vi "Geometric_Data.vi"() -> ()   [LabVIEW 2021]
panel:
  in  "cube length":dbl
  out "Volume 3":dbl
  out "L.S.A 2":dbl
  out "T.S.A 3":dbl
  out "On/Off":bool
  in  "stop 3":bool
  in  "circular cone arm length":dbl
  in  "circular cone radius":dbl
  in  "circular cone hieght":dbl
  out "Volume 2":dbl
  out "L.S.A":dbl
  out "T.S.A 2":dbl
  out "On/Off":bool
  in  "stop":bool
  in  "stop":bool
  out "On/Off":bool
  out "T.S.A":dbl
  out "L.S.A":dbl
  out "Volume":dbl
  in  "Cylinder Hieght":dbl
  in  "Cylinder Radius":dbl
  # "Cylinder"
  # "Circular Cone"
  # "Cube"
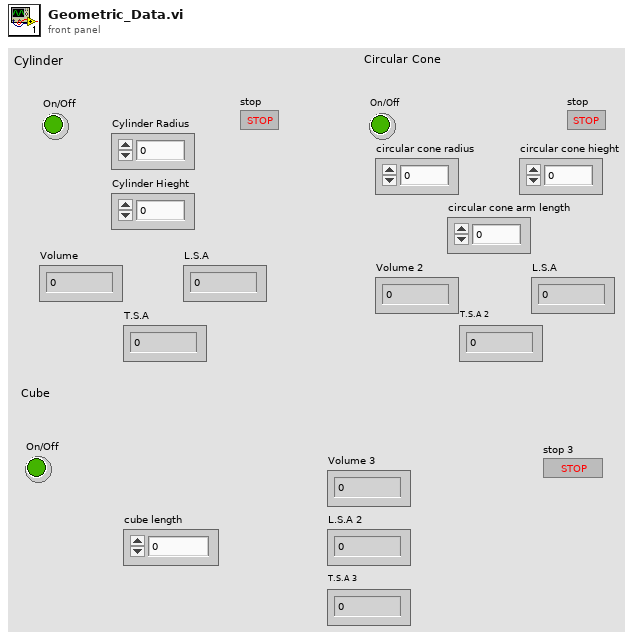
[diagram p1: front panel]
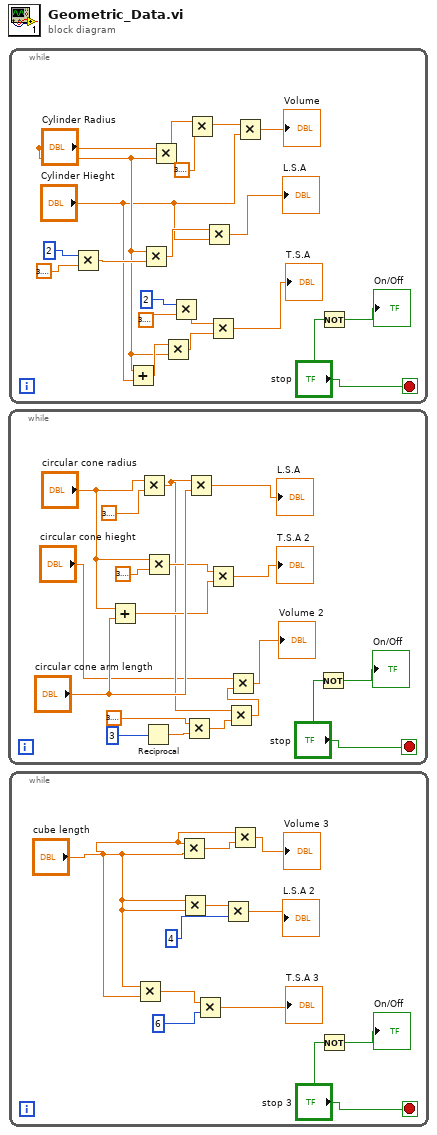
[diagram p0: block diagram]
diagram:
  n1 = while {
    stop <- "stop" stop-if-true
    n2 = Add(x="circular cone radius", y="circular cone arm length") -> (x+y=w10:dbl)
    n3 = Multiply(x="circular cone radius", y=3.141592653589793) -> (x*y=w4:dbl)
    n4 = Reciprocal(x=3) -> (1/x=w6:dbl)
    n5 = Multiply(x="circular cone radius", y=3.141592653589793) -> (x*y=w11:dbl)
    n6 = Multiply(x=3.141592653589793, y=w6) -> (x*y=w5:dbl)
    n7 = Multiply(x=w4, y="circular cone arm length") -> (x*y=→"L.S.A":dbl)
    n8 = Multiply(x=w11, y=w10) -> (x*y=→"T.S.A 2":dbl)
    n9 = Multiply(x=w4, y=w5) -> (x*y=w3:dbl)
    n10 = Multiply(x="circular cone hieght", y=w3) -> (x*y=→"Volume 2":dbl)
    n11 = Not(x="stop") -> (.not. x?=→"On/Off":bool)
  }
  n12 = while {
    stop <- "stop" stop-if-true
    n13 = Multiply(x=2, y=3.141592653589793) -> (x*y=w33:dbl)
    n14 = Add(x="Cylinder Radius", y="Cylinder Hieght") -> (x+y=w30:dbl)
    n15 = Multiply(x="Cylinder Radius", y=w33) -> (x*y=w32:dbl)
    n16 = Multiply(x="Cylinder Radius", y="Cylinder Radius") -> (x*y=w37:dbl)
    n17 = Multiply(x=w30, y="Cylinder Radius") -> (x*y=w25:dbl)
    n18 = Multiply(x=2, y=3.141592653589793) -> (x*y=w26:dbl)
    n19 = Multiply(x=w37, y=3.141592653589793) -> (x*y=w20:dbl)
    n20 = Multiply(x=w32, y="Cylinder Hieght") -> (x*y=→"L.S.A":dbl)
    n21 = Multiply(x=w26, y=w25) -> (x*y=→"T.S.A":dbl)
    n22 = Multiply(x=w20, y="Cylinder Hieght") -> (x*y=→"Volume":dbl)
    n23 = Not(x="stop") -> (.not. x?=→"On/Off":bool)
  }
  n24 = while {
    stop <- "stop 3" stop-if-true
    n25 = Multiply(x="cube length", y="cube length") -> (x*y=w39:dbl)
    n26 = Multiply(x="cube length", y="cube length") -> (x*y=w46:dbl)
    n27 = Multiply(x="cube length", y="cube length") -> (x*y=w44:dbl)
    n28 = Multiply(x=w39, y=6) -> (x*y=→"T.S.A 3":dbl)
    n29 = Multiply(x=w44, y=4) -> (x*y=→"L.S.A 2":dbl)
    n30 = Multiply(x="cube length", y=w46) -> (x*y=→"Volume 3":dbl)
    n31 = Not(x="stop 3") -> (.not. x?=→"On/Off":bool)
  }
